vi "IsGCodeExists.vi"(6 "error in (no error)":errorcluster, 8 "Destination Directory":path, 9 "VI (in)":refnum<vi>) -> (0 "error out":errorcluster, 1 "file or folder exists?":bool, 2 "VI Folder":path, 3 "VI (out)":refnum<vi>)   [LabVIEW 2017]
doc: "IsGCodeExists checks if GCode is already generated for VI\nThis is done by checking if a folder has been generated for given VI"
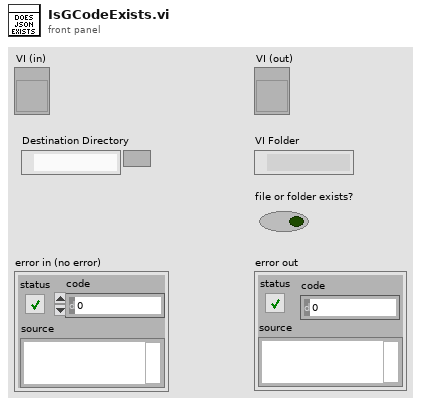
[diagram p1: front panel]
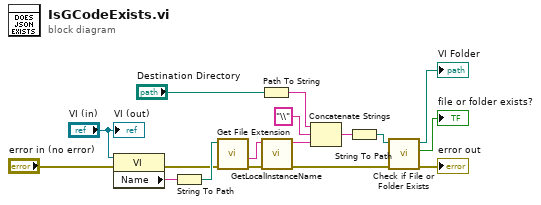
[diagram p0: block diagram]
diagram:
  n1 = property class="VI"(reference="VI (in)", error in="error in (no error)") -> (error out=w3:errorcluster, "Name"=w5:string)  [unwired: 1 out]
  n2 = String To Path(string=w5) -> (path=w4:path)
  n3 = call <vilib>:"Get File Extension.vi"("error in (no error)"=w3, "file"=w4) -> ("error out"=w2:errorcluster, "filename without extension"=w1:string)  [unwired: 5 in, 3 out]
  n4 = Path To String(path="Destination Directory") -> (string=w17:string)
  n5 = call "GetLocalInstanceName.vi"("error in (no error)"=w2, "result string in"=w1) -> ("error out"=w7:errorcluster, "result string out"=w6:string)  [unwired: 8 in]
  n6 = Concatenate Strings(w17, "\\" ("string"), w6) -> (w11:string)
  n7 = String To Path(string=w11) -> (path=w14:path)
  n8 = call <vilib>:"Check if File or Folder Exists.vi"("error in (no error)"=w7, "path"=w14) -> ("error out"=→"error out":errorcluster, "file or folder exists?"=→"file or folder exists?":bool, "dup path"=→"VI Folder":path)  [unwired: 7 in]
  "VI (out)" <- "VI (in)"
